vi "UDP_noinit.vi"(4 "connection ID":refnum<k16>, 5 "In":u8=255 format="%.0x", 6 "timeout ms (2000)":i32=2000, 7 "error in (no error)":errorcluster, 8 "Read (TRUE)":bool, 9 "Address":u32=64 format="%.0x", 10 "IP address":string="192.168.10.20") -> (0 "error out":errorcluster={"status"=TRUE, "code"=56, "source"="UDP Read in UDP.vi->flash.vi"}, 1 "Out":u8 format="%.0x", 2 "received string":string)   [LabVIEW 2017]
panel:
  out "字符串":string
  # "FFC0 0001 0000 0008"
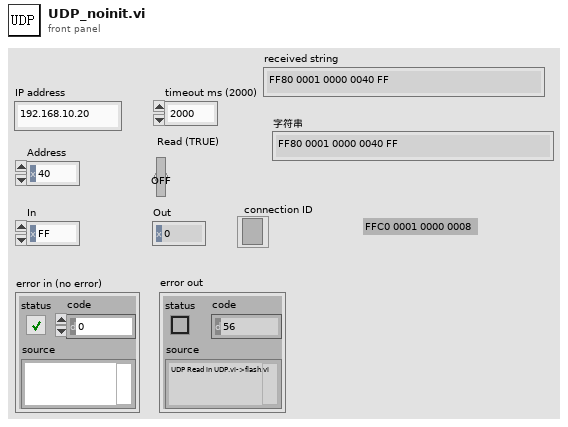
[diagram p1: front panel]
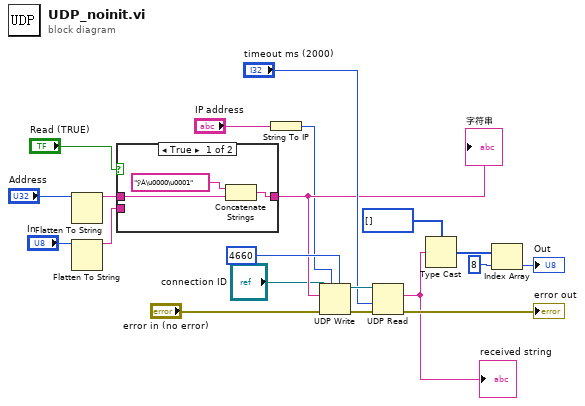
[diagram p0: block diagram]
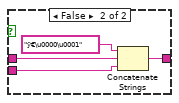
[diagram p2: hidden frame]
diagram:
  n1 = Flatten To String(anything="Address") -> (data string=w13:string)  [unwired: 3 in, 2 out]
  n2 = Flatten To String(anything="In") -> (data string=w11:string)  [unwired: 3 in, 2 out]
  n3 = case shown="True" "Read (TRUE)" {
    tunnel: [w22 w26] -> w15
    tunnel: w13 -> [w21 w25]
    tunnel: w11 -> [_ w24]
    frame True {
      n4 = Concatenate Strings("ÿÀ\u0000\u0001" ("initial string"), w21) -> (w22:string)
    }
    frame False {
      n5 = Concatenate Strings("ÿ€\u0000\u0001" ("initial string"), w25, w24) -> (w26:string)
    }
  }
  "字符串" <- w15
  n6 = String To IP(1:"IP address") -> (0:w5:u32)
  n7 = UDP Write(address=w5, port or service name=u16 4660 ("UDP port"), connection ID="connection ID", data in=w15, 8:"error in (no error)") -> (error out=w17:errorcluster, 3:w18:refnum<k16>)  [unwired: 1 in]
  n8 = UDP Read(connection ID=w18, timeout ms (25000)="timeout ms (2000)", 8:w17) -> (data out=w1:string, error out=→"error out":errorcluster)  [unwired: 4 out]
  "received string" <- w1
  n9 = Type Cast(type=u8[] [], x=w1) -> (*(type *) &x=w8:u8[])
  n10 = Index Array(array=w8, index=8) -> (element=→"Out":u8)
